vi "Calibrate Button Speed 2 Ticks (uSMC).vi"(1 "Speed (Full Step/Sec)":u16) -> (0 "Ticks":u16)   [LabVIEW 2010, in "SignalWriterMH110203USBStepperMotor.lvclass"]
uses:
  SignalWriterMH110203USBStepperMotor.lvclass
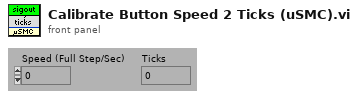
[diagram p1: front panel]
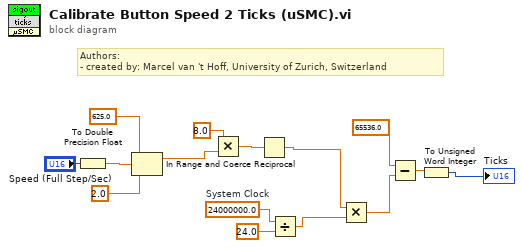
[diagram p0: block diagram]
diagram:
  w15 = 24000000.0  # System Clock
  # "Authors: \n- created by: Marcel van 't Hoff, University of Zurich, Switzerland"
  n1 = To Double Precision Float(number="Speed (Full Step/Sec)") -> (double precision float=w1:dbl)
  n2 = In Range and Coerce(upper limit=625.0, x=w1, lower limit=2.0) -> (coerced(x)=w4:dbl)  [unwired: 1 out]
  n3 = Multiply(x=8.0, y=w4) -> (x*y=w6:dbl)
  n4 = Reciprocal(x=w6) -> (1/x=w7:dbl)
  n5 = Divide(x=w15, y=24.0) -> (x/y=w9:dbl)
  n6 = Multiply(x=w7, y=w9) -> (x*y=w12:dbl)
  n7 = Subtract(x=65536.0, y=w12) -> (x-y=w11:dbl)
  n8 = To Unsigned Word Integer(number=w11) -> (unsigned 16bit integer=→"Ticks":u16)
